vi "rad_Get Second Image Info.vi"(5 "Password":string, 6 "Operation":T3, 7 "Comparison Image Path":path, 8 "error in (no error)":errorcluster, 9 "TempFolder Path":path, 10 "RT Target IP":string, 11 "Target settings in":T1={"Hostname"="", "Serial number"="", "Product name"="", "Product code"=0, "System status"="", "Credential type"=enum."None/Unlocked", "User added?"=FALSE, "Primary NIC"={"MAC address"="", "IP Address Request Mode"=2, "IP address"="", "Subnet mask"="", "Gateway"="", "DNS server"=""}} {"Primary NIC"."IP Address Request Mode" items=["Static"=1, "DHCP/Link-Local"=2, "Link-Local Only"=4, "DHCP Only"=8]}) -> (0 "error out":errorcluster, 1 "AppImage Properties":T4, 2 "Unzipped App Image Folder Path":path, 3 "Target settings out":T1={"Hostname"="", "Serial number"="", "Product name"="", "Product code"=0, "System status"="", "Credential type"=enum."None/Unlocked", "User added?"=FALSE, "Primary NIC"={"MAC address"="", "IP Address Request Mode"=2, "IP address"="", "Subnet mask"="", "Gateway"="", "DNS server"=""}} {"Primary NIC"."IP Address Request Mode" items=["Static"=1, "DHCP/Link-Local"=2, "Link-Local Only"=4, "DHCP Only"=8]})   [LabVIEW 2020]
uses:
  App Images/TypeDefs/rad_FPGA Flash Properties.ctl
  App Images/TypeDefs/rad_FPGA Properties.ctl
  App Images/TypeDefs/rad_Application Image Properties.ctl
  TypeDefs/rad_Comparison Modes.ctl
  Targets/TypeDefs/rad_Target Information.ctl
  Targets/TypeDefs/rad_Target Network Settings.ctl
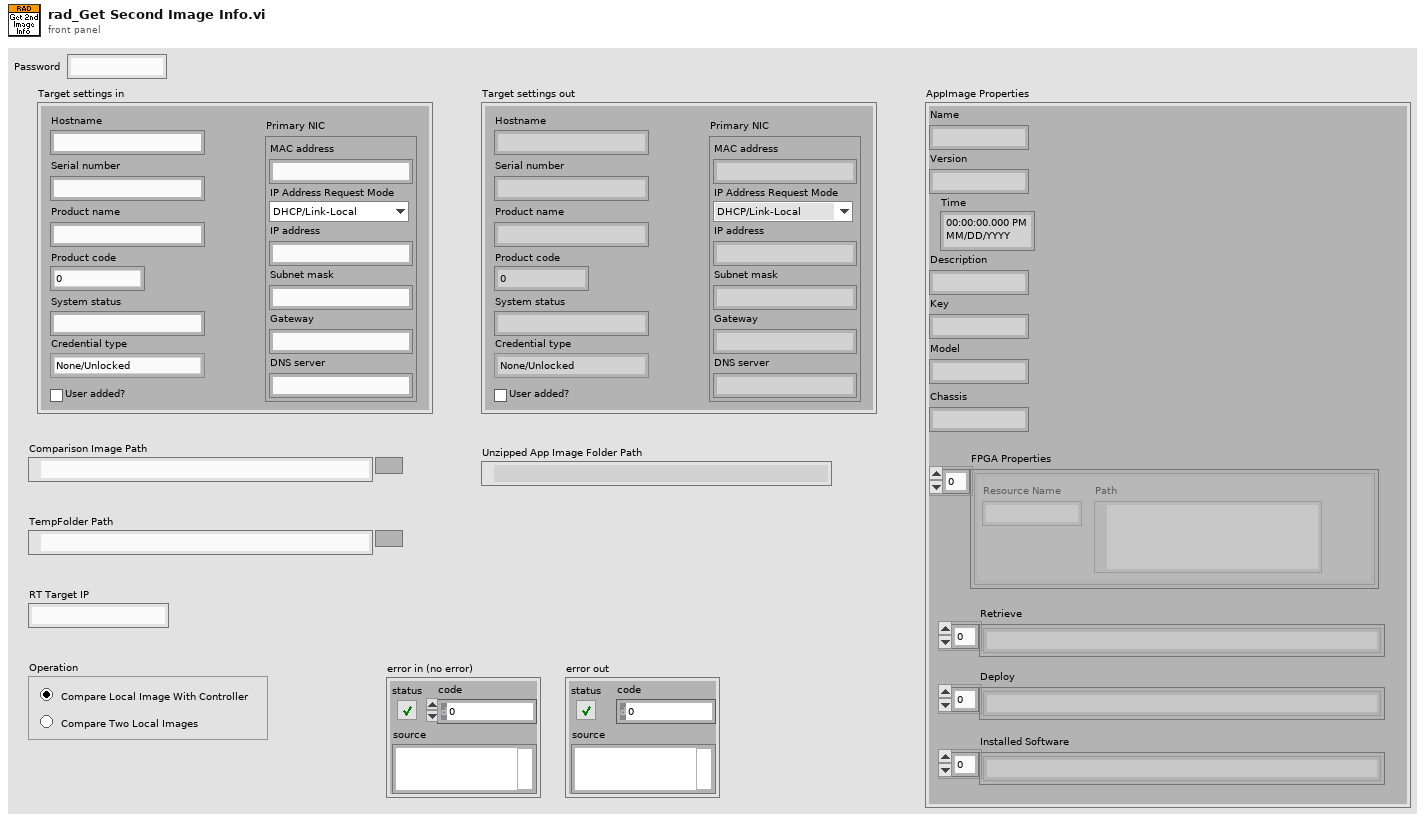
[diagram p1: front panel]
types:
  T1 = typedef "rad_Target Information.ctl" = cluster{"Hostname":string, "Serial number":string, "Product name":string, "Product code":i32, "System status":string, "Credential type":enum16{"None/Unlocked", "FTP Password", "NIAuth Credentials"}, "User added?":bool, "Primary NIC":T2}
  T2 = typedef "rad_Target Network Settings.ctl" = cluster{"MAC address":string, "IP Address Request Mode":i32, "IP address":string, "Subnet mask":string, "Gateway":string, "DNS server":string}
  T3 = typedef "rad_Comparison Modes.ctl" = enum32{"Compare Local Image With Controller", "Compare Two Local Images"}
  T4 = typedef "rad_Application Image Properties.ctl" = cluster{"Name":string, "Version":string, "Time":timestamp, "Description":string, "Key":string, "Chassis":string, "FPGA Properties":T5, "Model":string, "Retrieve":string[], "Deploy":string[], "Installed Software":string[]}
  T5 = typedef "rad_FPGA Properties.ctl" = T6[]
  T6 = typedef "rad_FPGA Flash Properties.ctl" = cluster{"Resource Name":string, "Path":path}
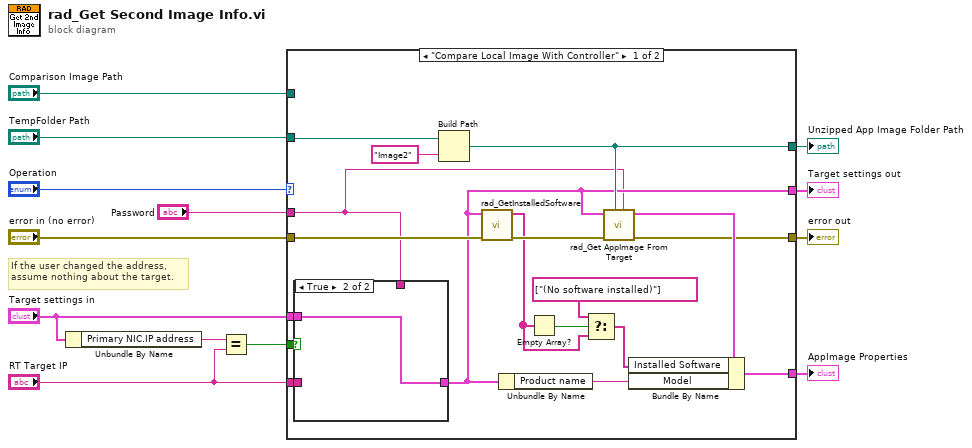
[diagram p0: block diagram]
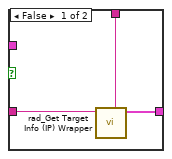
[diagram p2: hidden frame]
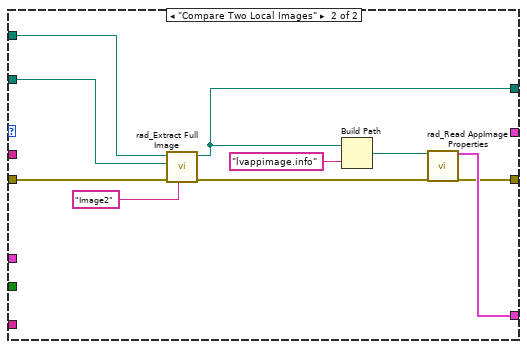
[diagram p3: hidden frame]
diagram:
  # "If the user changed the address,\nassume nothing about the target."
  n1 = Unbundle By Name("Target settings in") -> ("Primary NIC.IP address"=w6:string)
  n2 = Equal?(x=w6, y="RT Target IP") -> (x = y?=w7:bool)
  n3 = case shown="\"Compare Local Image With Controller\"" "Operation" {
    tunnel: [w20 w37] -> w12
    tunnel: "error in (no error)" -> [w22 w43]
    tunnel: [w26 w40] -> w3
    tunnel: "TempFolder Path" -> [w30 w45]
    tunnel: "Target settings in" -> [w28 _]
    tunnel: w7 -> [w29 _]
    tunnel: "RT Target IP" -> [w27 _]
    tunnel: [w25 w38] -> w11
    tunnel: "Comparison Image Path" -> [_ w36]
    tunnel: [w19 _] -> w2
    tunnel: "Password" -> [w14 _]
    frame "Compare Local Image With Controller" {
      n4 = case shown="True" w29 {
        tunnel: w28 -> [_ w35]
        tunnel: [w33 w35] -> w19
        tunnel: w27 -> [w34 _]
        tunnel: w14 -> [w32 _]
        frame False {
          n5 = call "rad_Get Target Info (IP) Wrapper.vi"("Password"=w32, "target address"=w34) -> ("Target settings"=w33:T1)  [unwired: 8 in, 1 out]
        }
        frame True {
        }
      }
      n6 = Build Path(base path=w30, name or relative path="Image2") -> (appended path=w26:path)
      n7 = call "rad_GetInstalledSoftware.vi"("error in (no error)"=w22, "Target settings"=w19) -> ("error out"=w21:errorcluster, "installedSoftware"=w17:string[])  [unwired: 8 in]
      n8 = Unbundle By Name(w19) -> ("Product name"=w24:string)
      n9 = Empty Array?(array=w17) -> (empty?=w18:bool)
      n10 = Select(t=string[] ["(No software installed)"], s=w18, f=w17) -> (s? t:f=w16:string[])
      n11 = call "rad_Get AppImage From Target.vi"("password"=w14, "Temp Folder"=w26, "error in (no error)"=w21, "Target settings"=w19) -> ("error out"=w20:errorcluster, "AppImage Properties"=w23:T4)  [unwired: 5 in, 1 out]
      n12 = Bundle By Name(cluster=w23, "Installed Software"=w16, "Model"=w24) -> (w25:T4)
    }
    frame "Compare Two Local Images" {
      n13 = call "rad_Extract Full Image.vi"("Subfolder (lvappimage.contents)"="Image2" ("name or relative path"), "error in (no error)"=w43, "App Image Temp Folder"=w45, "Zipped App Image File Path"=w36) -> ("error out"=w39:errorcluster, "Unzipped App Image Folder Path"=w40:path)  [unwired: 6 in]
      n14 = Build Path(base path=w40, name or relative path="lvappimage.info") -> (appended path=w42:path)
      n15 = call "rad_Read AppImage Properties.vi"("AppImage Properties Path"=w42, "error in (no error)"=w39) -> ("AppImage Properties"=w38:T4, "error out"=w37:errorcluster)  [unwired: 12 in, 4 out]
    }
  }
  "error out" <- w12
  "AppImage Properties" <- w11
  "Unzipped App Image Folder Path" <- w3
  "Target settings out" <- w2
